vi "十六进制U16转ASCII字符串 (子VI).vi"(11 "十六进制数值":u16 format="%xH") -> (3 "ASCII字符串输出":string)   [LabVIEW 2016, in "环境动力监测库.lvlib" / "空调库.lvlib"]
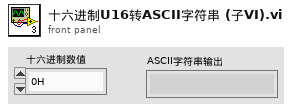
[diagram p1: front panel]
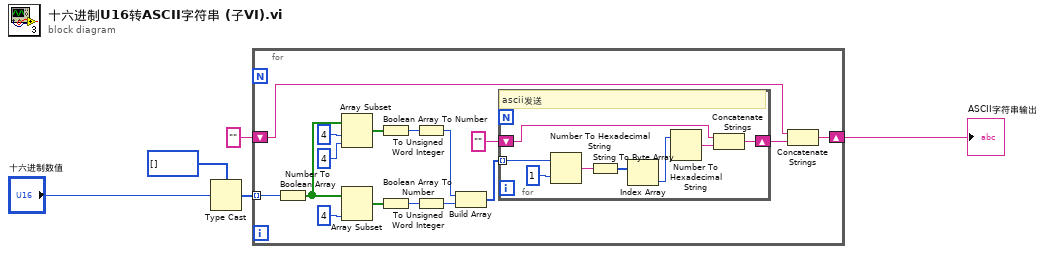
[diagram p0: block diagram]
diagram:
  n1 = Type Cast(type=u8[] [] ("无符号字节数组 2"), x="十六进制数值") -> (*(type *) &x=w3:u8[])
  n2 = for {
    tunnel: w3 -> [w9] mode=indexing
    shift-right: [w6] -> w1
    shift-left: "" -> [w8]
    n3 = Number To Boolean Array(number=w9) -> (Boolean array=w19:bool[])
    n4 = Array Subset(array=w19, index=4 ("索引"), length=4 ("长度")) -> (w16:bool[])
    n5 = Array Subset(array=w19, length=4 ("长度")) -> (w17:bool[])  [unwired: 1 in]
    n6 = Boolean Array To Number(Boolean array=w16) -> (number=w14:u32)
    n7 = Boolean Array To Number(Boolean array=w17) -> (number=w15:u32)
    n8 = To Unsigned Word Integer(number=w14) -> (unsigned 16bit integer=w12:u16)
    n9 = To Unsigned Word Integer(number=w15) -> (unsigned 16bit integer=w13:u16)
    n10 = Build Array(w12, w13) -> (w10:u16[])
    n11 = for {
      tunnel: w10 -> [w29] mode=indexing
      shift-right: [w24] -> w7
      shift-left: "" -> [w25]
      # "ascii发送"
      n12 = Number To Hexadecimal String(1:i16 1 ("宽度(-)"), 2:w29) -> (0:w23:string)
      n13 = String To Byte Array(string=w23) -> (unsigned byte array=w27:u8[])
      n14 = Index Array(array=w27) -> (element=w26:u8)  [unwired: 1 in]
      n15 = Number To Hexadecimal String(2:w26) -> (0:w22:string)  [unwired: 1 in]
      n16 = Concatenate Strings(w25, w22) -> (w24:string)
    }
    n17 = Concatenate Strings(w8, w7) -> (w6:string)
  }
  "ASCII字符串输出" <- w1
